vi "Get Temperature.vi"(6 "Channel":i32, 8 "error in (no error)":errorcluster, 11 "Instrument.TC.MNK in":refnum<class "Instrument.TC.MNK.lvclass">) -> (0 "error out":errorcluster, 1 "Status":string, 2 "Temperature (K)":dbl, 3 "Instrument.TC.MNK out":refnum<class "Instrument.TC.MNK.lvclass">, 4 "Finished?":bool)   [LabVIEW 2019, in "Instrument.TC.MNK.lvclass"]
uses:
  Instrument.TC.MNK.lvclass
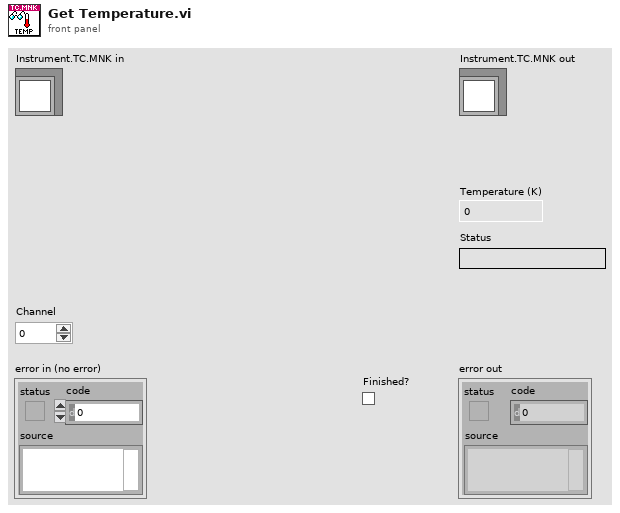
[diagram p1: front panel]
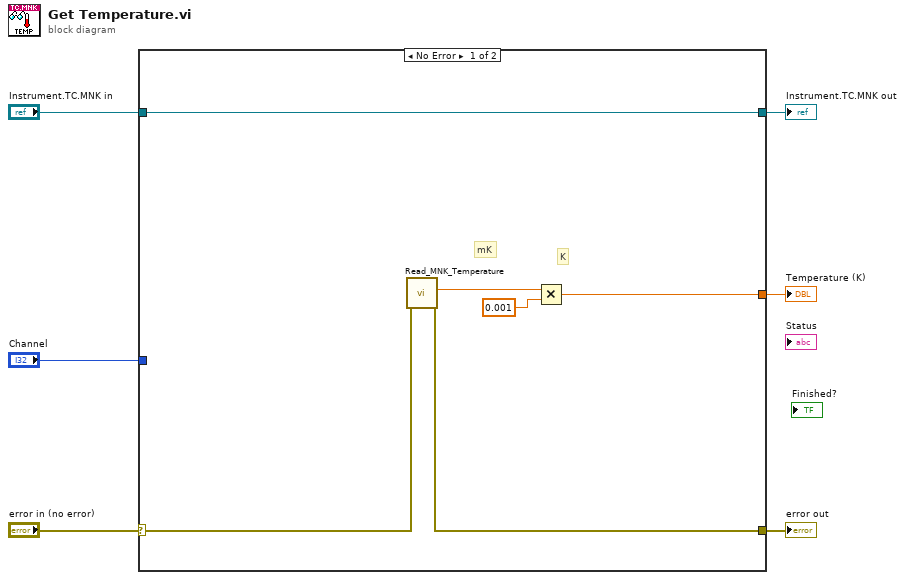
[diagram p0: block diagram]
diagram:
  n1 = case shown="No Error" "error in (no error)" {
    selector: "error in (no error)" -> [w10 w13]
    tunnel: [w9 w13] -> w5
    tunnel: [w12 w14] -> w4
    tunnel: "Instrument.TC.MNK in" -> [w12 w14]
    tunnel: [w7 _] -> w2
    tunnel: "Channel" -> [_ _]
    frame No Error {
      # "K"
      # "mK"
      n2 = call "Read_MNK_Temperature.vi"("Error in (no error)"=w10) -> ("Error out"=w9:errorcluster, "Temp"=w11:dbl)  [unwired: 9 in]
      n3 = Multiply(x=w11, y=0.001) -> (x*y=w7:dbl)
    }
    frame Error {
    }
  }
  "error out" <- w5
  "Instrument.TC.MNK out" <- w4
  "Temperature (K)" <- w2
